vi "VerifPreDCIR_P.vi"(8 "errin":errorcluster, 11 "VISA resource name":refnum<visa-resource-name>) -> (0 "errout":errorcluster caption="sortie d'erreur", 1 "Actual Current Level (A)":dbl format="%.2g", 2 "Actual Voltage Level (V)":dbl format="%.2g", 3 "V>10 ?":bool)   [LabVIEW 2020]
uses:
  5f35586e-bf77-4ad9-b645-b9e33e4f06e5.vi
  <instrlib>/IT6000C/IT6000C.lvlib
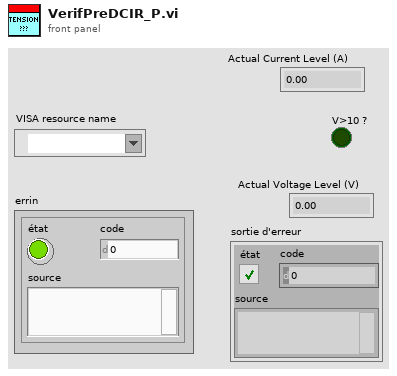
[diagram p1: front panel]
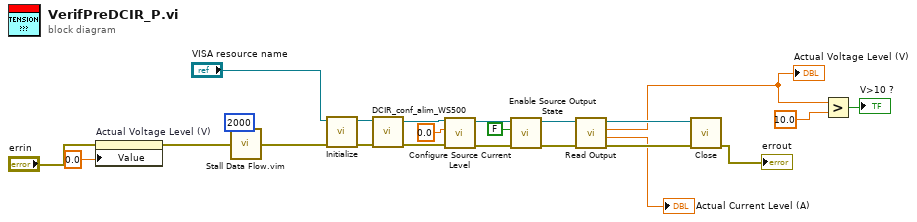
[diagram p0: block diagram]
diagram:
  n1 = property on="Actual Voltage Level (V)" class="DigNum (strict)"(error in="errin", "Value"=0.0 ("Actual Voltage Level (V)")) -> (error out=w6:errorcluster)  [unwired: 1 in, 1 out]
  n2 = call "Stall Data Flow.vim"("value in"=w6, "milliseconds to wait"=u32 2000) -> ("value out"=w10:errorcluster)  [unwired: 1 out]
  n3 = call <instrlib>:"Initialize.vi"("error in (no error)"=w10, "VISA resource name"="VISA resource name") -> ("error out"=w9:errorcluster, "VISA resource name out"=w11:refnum<visa-resource-name>)  [unwired: 8 in]
  n4 = call "DCIR_conf_alim_WS500.vi"("ErrIN"=w9, "VISAin"=w11) -> ("ErrOUT"=w22:errorcluster, "VisaOUT"=w21:refnum<visa-resource-name>)  [unwired: 8 in]
  n5 = call <instrlib>:"Configure Source Current Level.vi"("error in (no error)"=w22, "Value(0)"=0.0, "VISA resource name"=w21) -> ("error out"=w20:errorcluster, "VISA resource name out"=w19:refnum<visa-resource-name>)  [unwired: 7 in]
  n6 = call <instrlib>:"Enable Source Output State.vi"("error in (no error)"=w20, "Enable(True)"=FALSE, "VISA resource name"=w19) -> ("error out"=w16:errorcluster, "VISA resource name out"=w15:refnum<visa-resource-name>)  [unwired: 7 in]
  n7 = call <instrlib>:"Read Output.vi"("error in (no error)"=w16, "VISA resource name"=w15) -> ("error out"=w14:errorcluster, "Actual Current Level (A)"=→"Actual Current Level (A)":dbl, "Actual Voltage Level (V)"=w5:dbl, "VISA resource name out"=w13:refnum<visa-resource-name>)  [unwired: 6 in]
  "Actual Voltage Level (V)" <- w5
  n8 = call <instrlib>:"Close.vi"("error in (no error)"=w14, "VISA resource name"=w13) -> ("error out"=→"errout":errorcluster)  [unwired: 9 in]
  n9 = Greater?(x=w5, y=10.0) -> (0:→"V>10 ?":bool)
